vi "BoxExecute.vi"(8 "error in (no error)":errorcluster) -> (0 "error out":errorcluster)   [LabVIEW 2023]
uses:
  <vilib>/Rock Robotics/WPI/ThirdParty/REV Robotics/REVLib/Typedef/Spark MAX Control Type.ctl
  BoxStatesEnum.ctl
  BoxNoteState.ctl
  <vilib>/Rock Robotics/WPI/ThirdParty/JAS_Junk/TrajLib/TypeDef/PID_ERROR_TOLERANCE.ctl
  <vilib>/Rock Robotics/WPI/ThirdParty/JAS_Junk/TrajLib/LinearFilter_LP_BW1_Execute.vi
  <vilib>/Rock Robotics/WPI/ThirdParty/JAS_Junk/TrajLib/VI/BoolCmd_Recv_Internal.vi
  <vilib>/Rock Robotics/WPI/ThirdParty/JAS_Junk/TrajLib/PIDController_AtSetpoint.vi
  <vilib>/Rock Robotics/WPI/ThirdParty/JAS_Junk/TrajLib/PIDController_SetPIDF.vi
  <vilib>/Rock Robotics/WPI/ThirdParty/JAS_Junk/TrajLib/PIDController_SetDerivativeFilter.vi
  <vilib>/Rock Robotics/WPI/ThirdParty/JAS_Junk/TrajLib/PIDController_SetIntegratorRange.vi
  <vilib>/Rock Robotics/WPI/ThirdParty/JAS_Junk/TrajLib/PIDController_SetTolerancePandV.vi
  <vilib>/Rock Robotics/WPI/ThirdParty/JAS_Junk/TrajLib/PIDController_DisableContinousInput.vi
  <vilib>/Rock Robotics/WPI/ThirdParty/JAS_Junk/TrajLib/PIDController_EnableContinousInput.vi
  <vilib>/Rock Robotics/WPI/ThirdParty/JAS_Junk/TrajLib/PIDController_Reset.vi
  <vilib>/Rock Robotics/WPI/ThirdParty/JAS_Junk/TrajLib/PIDController_New.vi
  <vilib>/Rock Robotics/WPI/ThirdParty/JAS_Junk/TrajLib/PIDController_SetOutputLimits.vi
  <vilib>/Rock Robotics/WPI/ThirdParty/JAS_Junk/TrajLib/VI/PIDController_SetIntegratorZone.vi
  <vilib>/Rock Robotics/WPI/ThirdParty/JAS_Junk/TrajLib/SimpleMotorFF_Calculate.vi
  <vilib>/Rock Robotics/WPI/ThirdParty/JAS_Junk/TrajLib/LinearFilter_ResetToValue.vi
  <vilib>/Rock Robotics/WPI/ThirdParty/JAS_Junk/TrajLib/LinearFilter_Calculate.vi
  <vilib>/Rock Robotics/WPI/ThirdParty/JAS_Junk/TrajLib/SlewRateLimiter_New.vi
  <vilib>/Rock Robotics/WPI/ThirdParty/JAS_Junk/TrajLib/SlewRateLimiter_Reset.vi
  <vilib>/Rock Robotics/WPI/ThirdParty/JAS_Junk/TrajLib/SlewRateLimiter_Calculate.vi
  <vilib>/Rock Robotics/WPI/ThirdParty/JAS_Junk/TrajLib/SlewRateLimiter_SetRate.vi
  <vilib>/Rock Robotics/WPI/ThirdParty/JAS_Junk/TrajLib/VI/BoolCmd_ObtainQueue.vi
  <vilib>/Rock Robotics/WPI/ThirdParty/JAS_Junk/TrajLib/PIDController_NewPeriod.vi
  <vilib>/Rock Robotics/WPI/ThirdParty/JAS_Junk/TrajLib/Util_GetTime.vi
  <vilib>/Rock Robotics/SystemInterfaces/NetworkCommunication/NetComm_UsageReport_report.vi
  <vilib>/Rock Robotics/WPI/ThirdParty/JAS_Junk/TrajLib/VI/Util_GetTime_U32.vi
  BoxGlobals.vi
  BoxNetworkingGlobal.vi
  <vilib>/Rock Robotics/WPI/ThirdParty/REV Robotics/REVLib/SubVI/Public/SPARK Get Encoder Status Velocity.vi
  <vilib>/Utility/semaphor.llb/Obtain Semaphore Reference.vi
  <vilib>/Rock Robotics/WPI/ThirdParty/JAS_Junk/TrajLib/Timer_Reset.vi
  <vilib>/Rock Robotics/WPI/ThirdParty/JAS_Junk/TrajLib/Timer_Start.vi
  <vilib>/Rock Robotics/WPI/ThirdParty/JAS_Junk/TrajLib/Timer_Stop.vi
  <vilib>/Rock Robotics/WPI/ThirdParty/JAS_Junk/TrajLib/LinearFilter_LowPassBW1.vi
  <vilib>/Rock Robotics/SystemInterfaces/Utilities/FPGA_UtilitiesRead LocalTime.vi
  <vilib>/Rock Robotics/WPI/ThirdParty/JAS_Junk/TrajLib/VI/Util_GetTime_U64.vi
  <vilib>/Rock Robotics/WPI/ThirdParty/JAS_Junk/TrajLib/Globals/Util_LibraryGlobals.vi
  <vilib>/Rock Robotics/WPI/ThirdParty/JAS_Junk/TrajLib/PIDController_AdvCalculate_FF_Sp_Pv.vi
  <vilib>/Rock Robotics/WPI/ThirdParty/JAS_Junk/TrajLib/Trajectory_Library.lvlib
panel:
  # "Click here to set min"
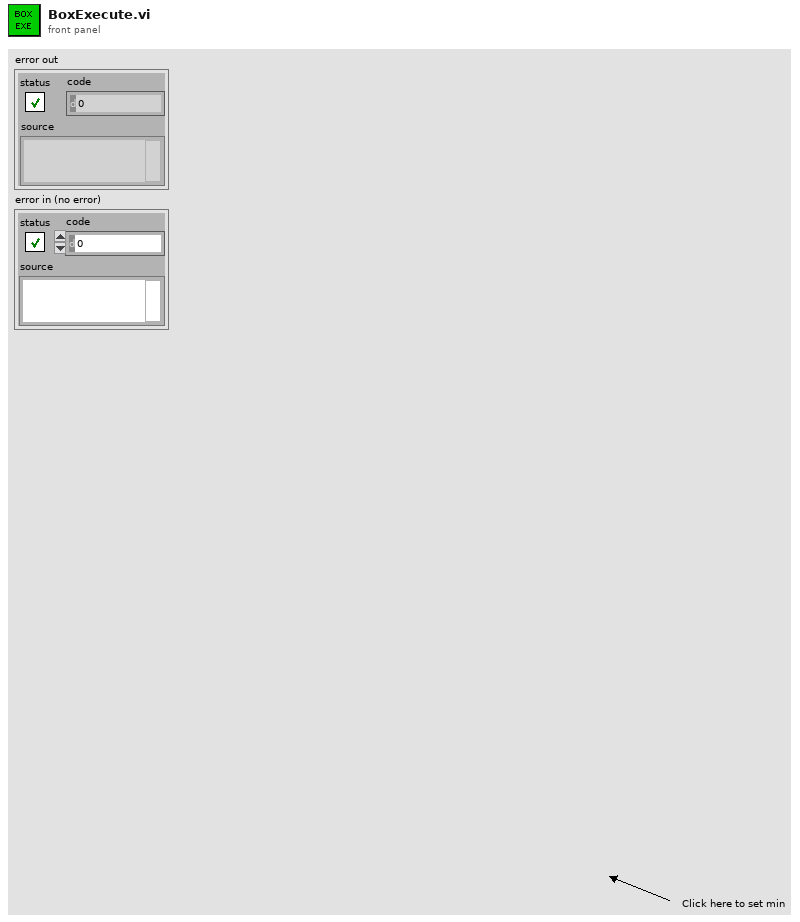
[diagram p1: front panel]
types:
  T1 = typedef "Spark MAX Control Type.ctl" = enum16{"Percent VBus", "Voltage", "Velocity", "Position", "Smart Motion", "Current", "Smart Velocity", "MAXMotion Position", "MAXMotion Velocity"}
  T2 = typedef "BoxStatesEnum.ctl" = enum16{"get input", "start shoot wheels", "up to speed?", "run intake", "have ring?", "stop intake and shooter", "start intake", "pick up ring or  _ sec?", "stop intake", "start source  intake", "pick up note?", "stop intake shooter", "shoot amp", "used note?", "stop amp intake", "initilization", "pre rev"}
  T3 = typedef "BoxNoteState.ctl" = enum16{"note in shooter wheels", "misaligned note", "no note", "have note"}
  T4 = typedef "Trajectory_Library.lvlib/PID_ERROR_TOLERANCE.ctl" = cluster{"PositionTolerance":dbl, "VelocityTolerance":dbl}
  T5 = typedef "WPI_DigitalInputDevRef.ctl" = cluster{"DevStatus":errorcluster, "DIO Channel":T6}
  T6 = typedef "FPGA_DIOChannel.ctl" = enum8{"DIO 0", "DIO 1", "DIO 2", "DIO 3", "DIO 4", "DIO 5", "DIO 6", "DIO 7", "DIO 8", "DIO 9", "DIO MXP 0", "DIO MXP 1", "DIO MXP 2", "DIO MXP 3", "DIO MXP 4", "DIO MXP 5", "DIO MXP 6", "DIO MXP 7", "DIO MXP 8", "DIO MXP 9", "DIO MXP 10", "DIO MXP 11", "DIO MXP 12", "DIO MXP 13", "DIO MXP 14", "DIO MXP 15", "SPI Port CS1", "SPI Port CS2", "SPI Port CS3", "SPI Port MISO", "SPI Port MOSI", "Invalid"}
  T7 = typedef "WPI_MotorControlDeviceRef.ctl" = cluster{"DeviceStatus":errorcluster, "Type":T8, "PWM":cluster{"PWM Channel":T9, "DeadBand":T10}, "CAN":cluster{"Device Number":u8, "SetOutput VI Ref":variant, "GetOutput VI Ref":variant, "Enable VI Ref":variant, "Disable VI Ref":variant, "Data":variant}, "Invert":bool, "DIO PWM":cluster{"PWM \"Enable\" Channel":T9, "DIOChannel":T6, "PWM Rate":dbl}}
  T8 = typedef "WPI_MotorControlType.ctl" = enum16{"PWM", "CAN", "DIO PWM"}
  T9 = typedef "FPGA_DIOPWMChannel.ctl" = enum8{"PWM 0", "PWM 1", "PWM 2", "PWM 3", "PWM 4", "PWM 5", "PWM 6", "PWM 7", "PWM 8", "PWM 9", "PWM MXP 0", "PWM MXP 1", "PWM MXP 2", "PWM MXP 3", "PWM MXP 4", "PWM MXP 5", "PWM MXP 6", "PWM MXP 7", "PWM MXP 8", "PWM MXP 9", "Invalid"}
  T10 = typedef "WPI_PWMDeadband.ctl" = cluster{"Name":string, "maxPositivePwm":i32, "minPositivePwm":i32, "centerPwm":i32, "maxNegativePwm":i32, "minNegativePwm":i32, "angularRange":u16}
  T11 = typedef "Trajectory_Library.lvlib/TIMER.ctl" = cluster{"StartTime":dbl, "Accumulated TIme":dbl, "Running":bool, "semaphore":T12}
  T12 = typedef "Semaphore RefNum" = refnum<k1>
  T13 = typedef "Trajectory_Library.lvlib/SIMPLE_MOTOR_FF.ctl" = cluster{"Ks":dbl, "Kv":dbl, "Ka":dbl, "KnInv":dbl}
  T14 = typedef "Trajectory_Library.lvlib/PID_ADV_LIMITS.ctl" = cluster{"MaxInput":dbl, "MinInput":dbl, "Continuous":bool, "MaxOutput":dbl, "MinOutput":dbl}
  T15 = typedef "Trajectory_Library.lvlib/PID_ADV_TUNING.ctl" = cluster{"Kf":dbl, "Kp":dbl, "Ki":dbl, "Kd":dbl, "MaximumIntegral":dbl, "MinimumIntegral":dbl, "Filter Derivative":bool, "IntegralZone":dbl}
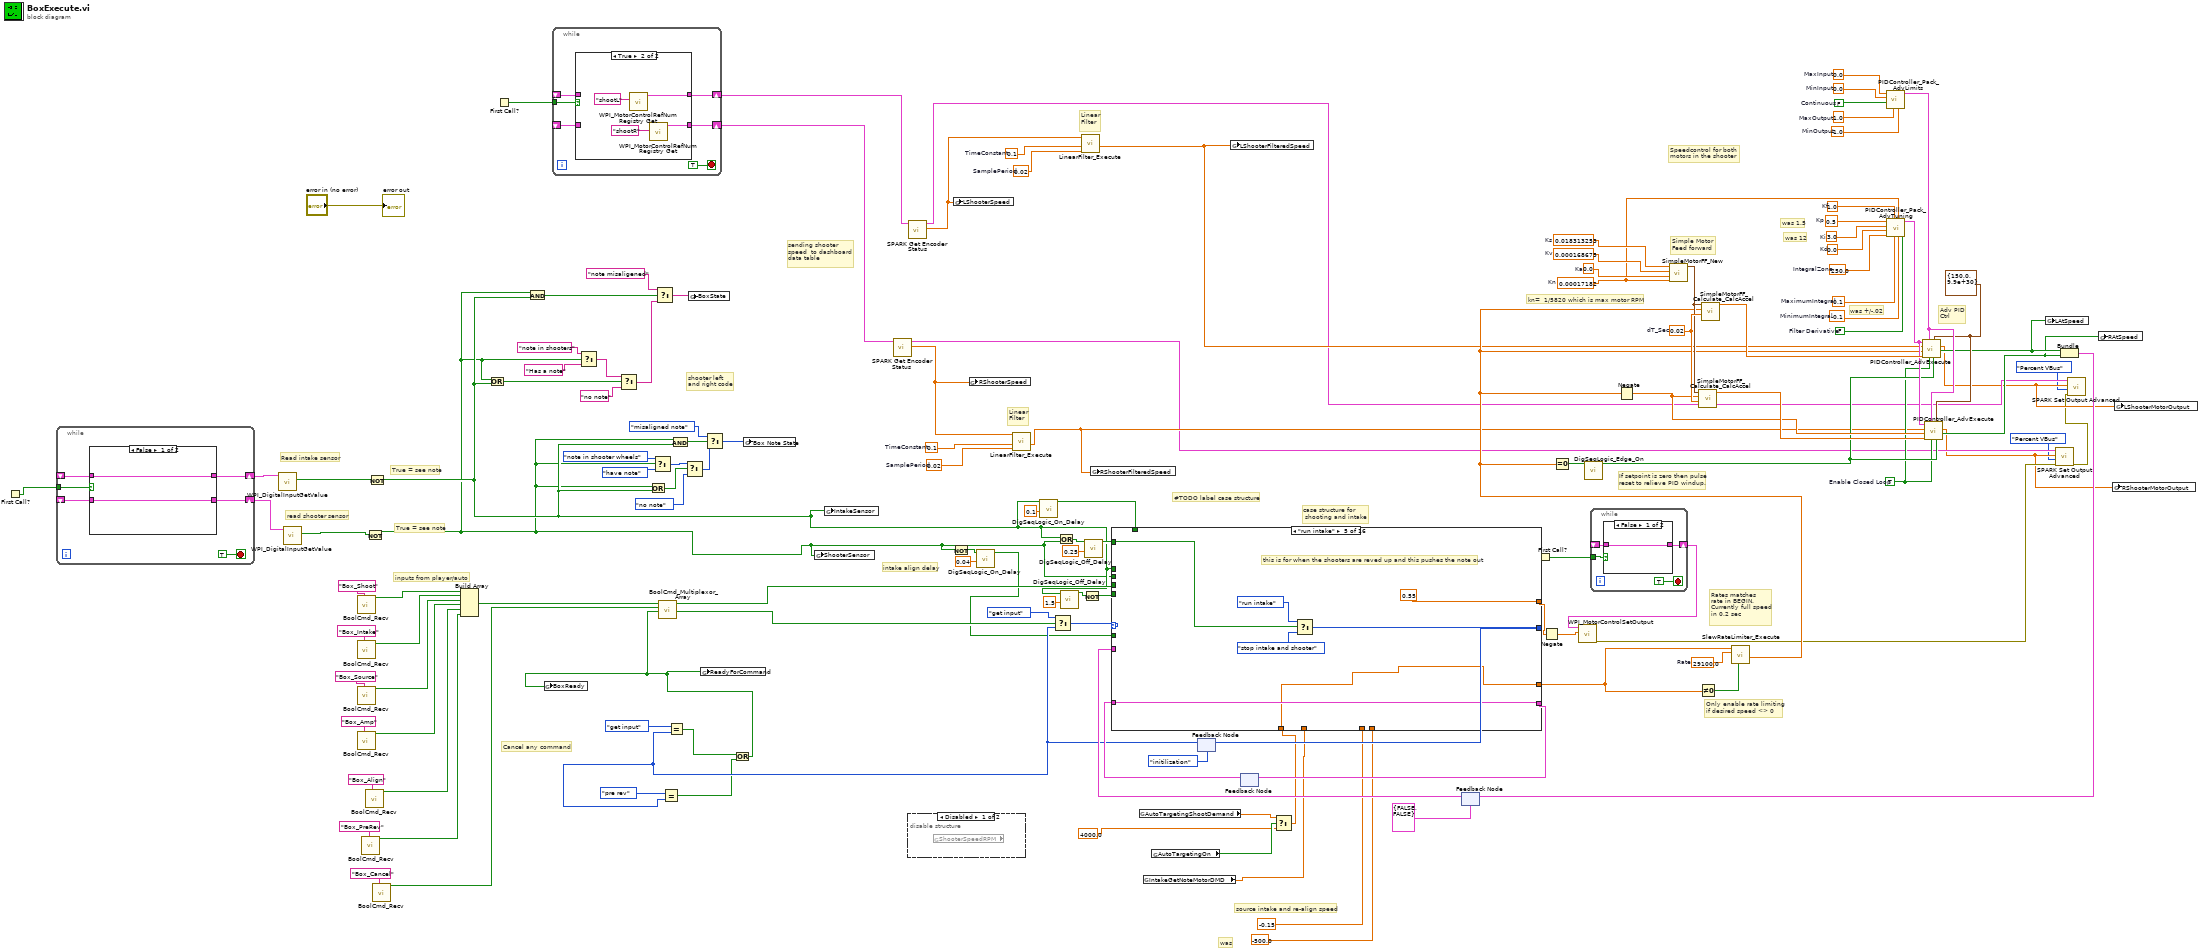
[diagram p0: block diagram]
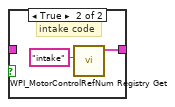
[diagram p3: hidden frame]
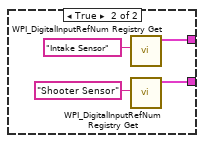
[diagram p4: hidden frame]
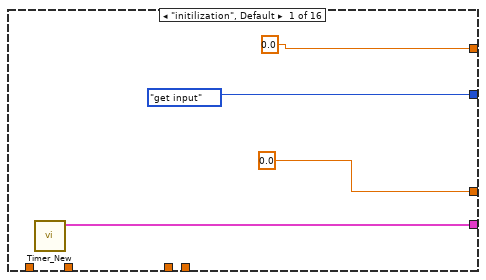
[diagram p6: hidden frame]
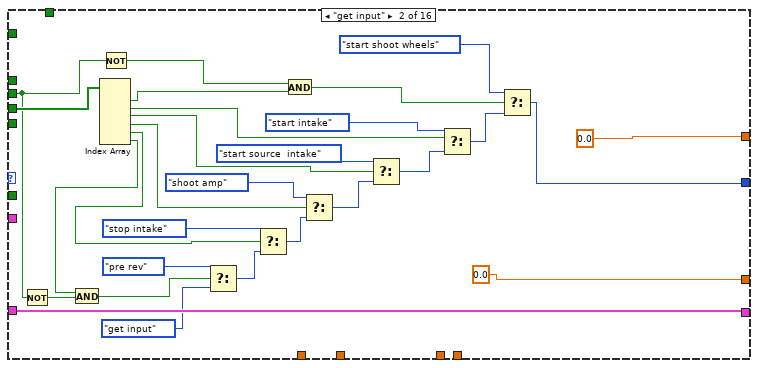
[diagram p7: hidden frame]
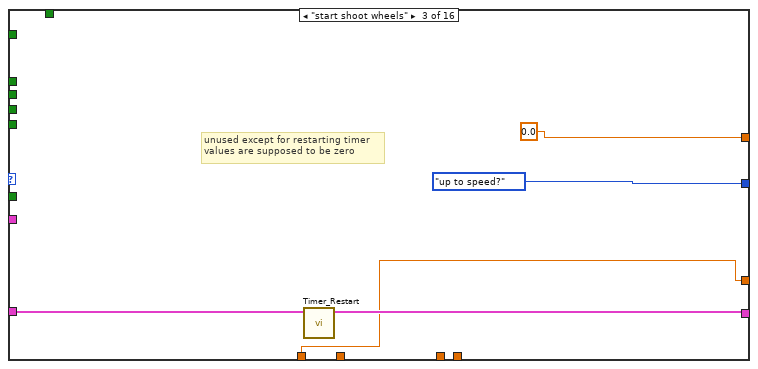
[diagram p8: hidden frame]
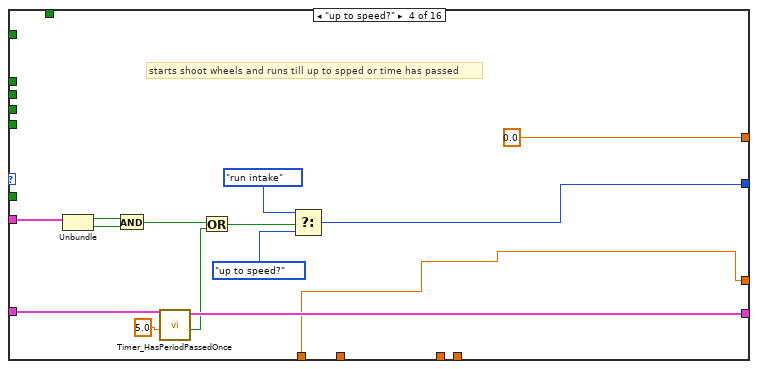
[diagram p9: hidden frame]
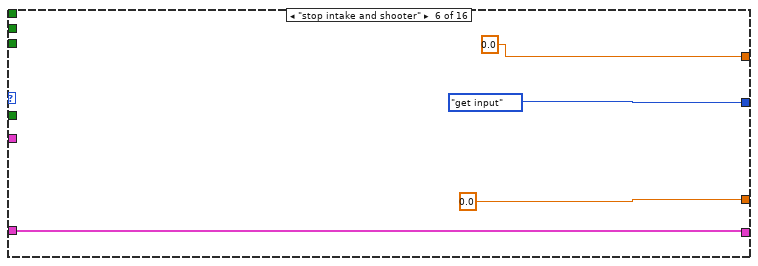
[diagram p10: hidden frame]
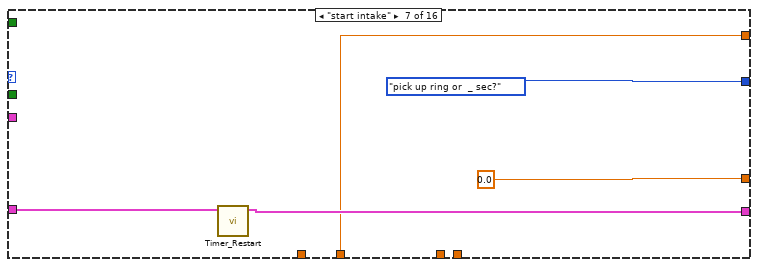
[diagram p11: hidden frame]
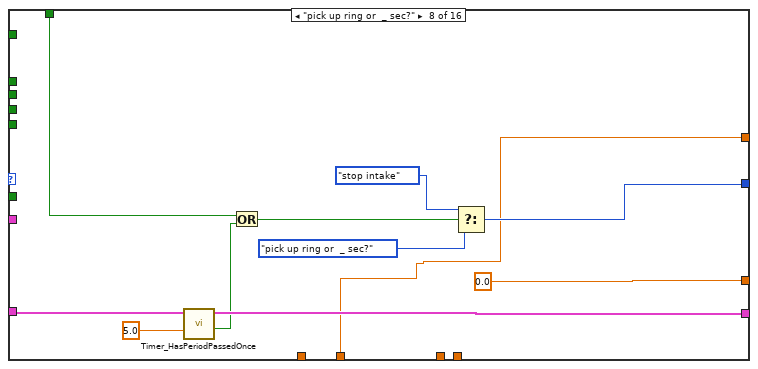
[diagram p12: hidden frame]
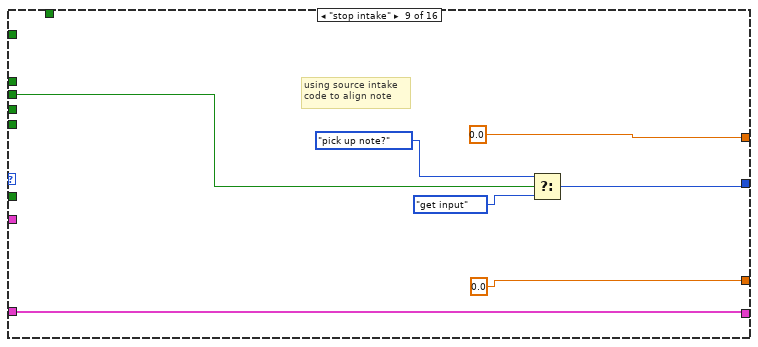
[diagram p13: hidden frame]
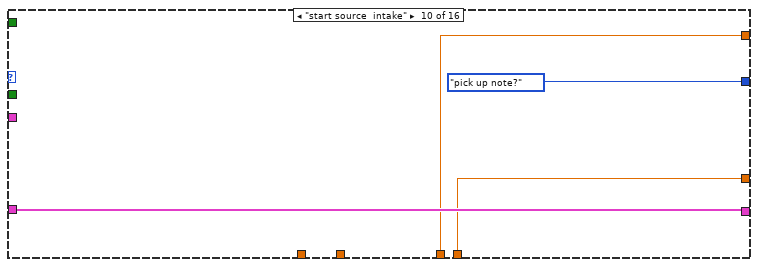
[diagram p14: hidden frame]
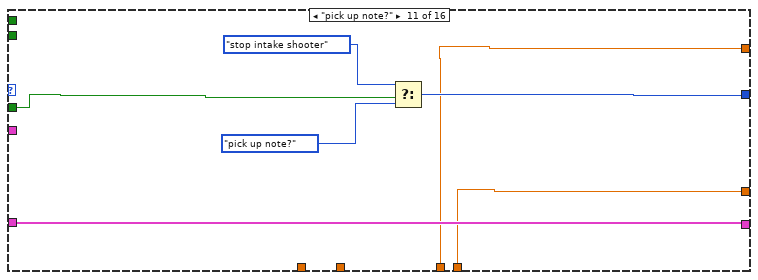
[diagram p15: hidden frame]
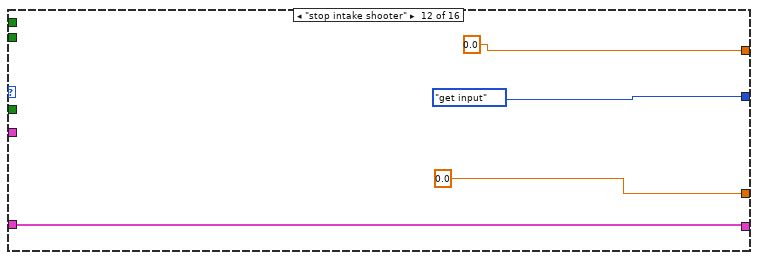
[diagram p16: hidden frame]
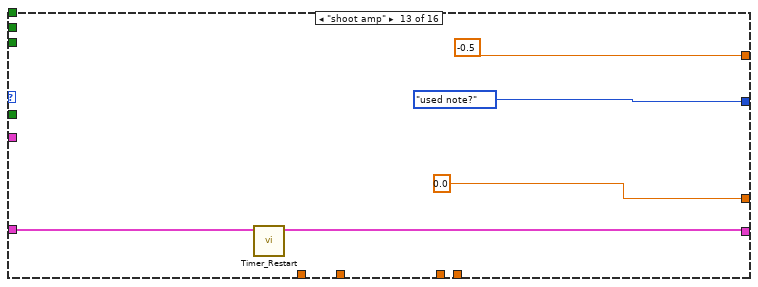
[diagram p17: hidden frame]
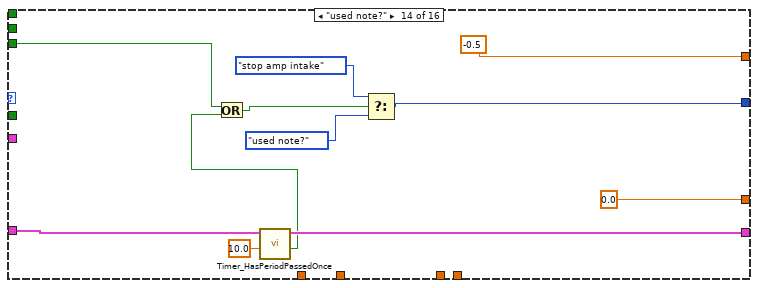
[diagram p18: hidden frame]
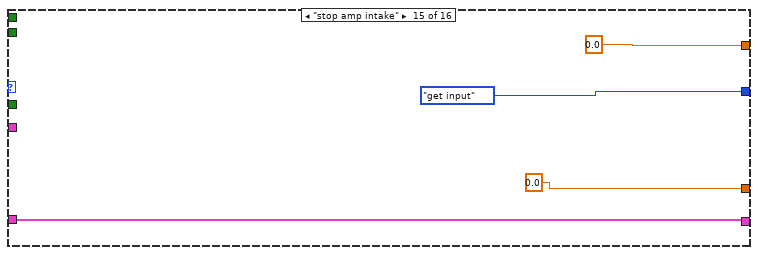
[diagram p19: hidden frame]
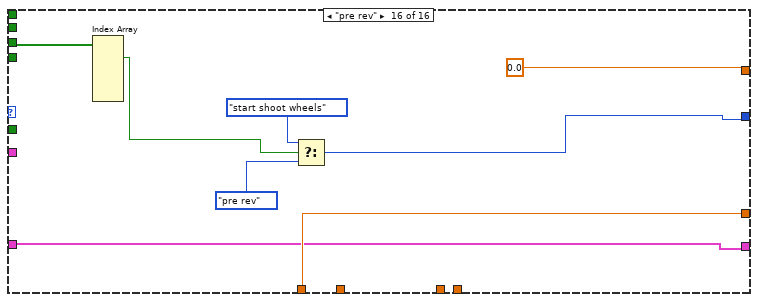
[diagram p20: hidden frame]
diagram:
  w21 = 250.0  # IntegralZone
  w50 = 29100.0  # Rate
  w12 = 0.02  # SamplePeriod
  w13 = 0.1  # TimeConstant
  w85 = 0.02  # SamplePeriod
  w9 = 0.1  # TimeConstant
  w47 = TRUE  # Enable Closed Loop
  w89 = T4 {"PositionTolerance"=150.0, "VelocityTolerance"=9.9e+30} ("PID Error Tolerance")
  w101 = 0.00017182  # Kn
  w104 = 0.018313253  # Ks
  w103 = 0.000168675  # Kv
  w102 = 0.0  # Ka
  w99 = 0.5  # Kp
  w98 = 3.0  # Ki
  w97 = 0.0  # Kd
  w100 = 1.0  # Kf
  w96 = 0.1  # MaximumIntegral
  w95 = -0.1  # MinimumIntegral
  w94 = FALSE  # Filter Derivative
  w108 = 0.0  # MinInput
  w107 = FALSE  # Continuous
  w106 = 1.0  # MaxOutput
  w105 = -1.0  # MinOutput
  w109 = 0.0  # MaxInput
  w93 = 0.02  # dT_Sec
  # "intake align delay"
  # "was"
  # "source intake and re-align speed"
  # "was 12"
  # "was 1.5"
  # "True = see note"
  # "True = see note"
  # "read shooter sensor"
  # "Read intake sensor"
  # "was +/-.02"
  # "If setpoint is zero then pulse\nreset to relieve PID windup."
  # "Rates matches\nrate in BEGIN.  \nCurrently full speed\nin 0.2 sec"
  # "Only enable rate limiting\nif desired speed <> 0"
  # "#TODO label case structure"
  # "inputs from player/auto"
  # "Linear\nFilter"
  # "Linear\nFilter"
  # "Speedcontrol for both \nmotors in the shooter"
  # "Simple Motor\nFeed forward"
  # "Adv PID\nCtrl"
  # "Cancel any command"
  # "kn=  1/5820 which is max motor RPM"
  # "case structure for\n shooting and intake"
  # "sending shooter \nspeed  to dashboard \ndata table"
  # "shooter left \nand right code"
  n1 = First Call?() -> (First Call?: T/F=w45:bool)
  n2 = while {
    tunnel: w45 -> [w137]
    shift-right: [w138] -> w113
    shift-left: _ -> [w136]
    shift-right: [w139] -> w114
    shift-left: _ -> [w135]
    stop <- TRUE stop-if-true
    n3 = case shown="False" w137 {
      tunnel: [w140 w145] -> w139
      tunnel: [w141 w144] -> w138
      tunnel: w136 -> [w141 _]
      tunnel: w135 -> [w140 _]
      frame False {
      }
      frame True {
        n4 = call <vilib>:"WPI_DigitalInputRefNum Registry Get.vi"("refnum name"="Intake Sensor") -> ("DigitalInputDevRef"=w144:T5)  [unwired: 9 in, 1 out]
        n5 = call <vilib>:"WPI_DigitalInputRefNum Registry Get.vi"("refnum name"="Shooter Sensor") -> ("DigitalInputDevRef"=w145:T5)  [unwired: 9 in, 1 out]
      }
    }
  }
  n6 = call <vilib>:"WPI_DigitalInputGetValue.vi"("DigitalInputDevRef"=w113) -> ("Value"=w74:bool)  [unwired: 8 in, 2 out]
  n7 = call <vilib>:"WPI_DigitalInputGetValue.vi"("DigitalInputDevRef"=w114) -> ("Value"=w73:bool)  [unwired: 8 in, 2 out]
  n8 = call <vilib>:"BoolCmd_Recv.vi"("Command Name"="Box_Shoot") -> ("New Request"=w124:bool)  [unwired: 9 in, 1 out]
  n9 = call <vilib>:"BoolCmd_Recv.vi"("Command Name"="Box_Intake") -> ("New Request"=w125:bool)  [unwired: 9 in, 1 out]
  n10 = call <vilib>:"BoolCmd_Recv.vi"("Command Name"="Box_Source") -> ("New Request"=w128:bool)  [unwired: 9 in, 1 out]
  n11 = call <vilib>:"BoolCmd_Recv.vi"("Command Name"="Box_Amp") -> ("New Request"=w129:bool)  [unwired: 9 in, 1 out]
  n12 = call <vilib>:"BoolCmd_Recv.vi"("Command Name"="Box_PreRev") -> ("New Request"=w38:bool)  [unwired: 9 in, 1 out]
  n13 = call <vilib>:"BoolCmd_Recv.vi"("Command Name"="Box_Align") -> ("New Request"=w53:bool)  [unwired: 9 in, 1 out]
  n14 = Not(x=w73) -> (.not. x?=w18:bool)
  n15 = Not(x=w74) -> (.not. x?=w30:bool)
  n16 = call <vilib>:"BoolCmd_Recv.vi"("Command Name"="Box_Cancel") -> ("New Request"=w122:bool)  [unwired: 9 in, 1 out]
  n17 = Build Array(w124, w125, w128, w129, w53, w38) -> (w123:bool[])
  n18 = Or(x=w18, y=w30) -> (x .or. y?=w81:bool)
  n19 = First Call?() -> (First Call?: T/F=w46:bool)
  n20 = And(x=w18, y=w30) -> (x .and. y?=w82:bool)
  n21 = while {
    tunnel: w46 -> [w149]
    shift-right: [w151] -> w15
    shift-left: _ -> [w147]
    shift-right: [w150] -> w11
    shift-left: _ -> [w146]
    stop <- TRUE stop-if-true
    n22 = case shown="True" w149 {
      tunnel: [w153 w155] -> w151
      tunnel: [w152 w154] -> w150
      tunnel: w147 -> [w153 _]
      tunnel: w146 -> [w152 _]
      frame False {
      }
      frame True {
        n23 = call <vilib>:"WPI_MotorControlRefNum Registry Get.vi"("refnum name"="shootL") -> ("MotorControlDevRef"=w155:T7)  [unwired: 9 in, 1 out]
        n24 = call <vilib>:"WPI_MotorControlRefNum Registry Get.vi"("refnum name"="shootR") -> ("MotorControlDevRef"=w154:T7)  [unwired: 9 in, 1 out]
      }
    }
  }
  n25 = Select(t="note in shooters", s=w18, f="Has a note") -> (s? t:f=w80:string)
  n26 = Select(t=w80, s=w81, f="no note") -> (s? t:f=w78:string)
  n27 = Or(x=w18, y=w30) -> (x .or. y?=w71:bool)
  n28 = Select(t=BoxNoteState."note in shooter wheels" ("Box Note State"), s=w18, f=BoxNoteState."have note" ("Box Note State")) -> (s? t:f=w70:T3)
  n29 = Select(t="note misaligened", s=w82, f=w78) -> (s? t:f=w29:string)
  n30 = And(x=w18, y=w30) -> (x .and. y?=w72:bool)
  n31 = Select(t=w70, s=w71, f=BoxNoteState."no note" ("Box Note State")) -> (s? t:f=w69:T3)
  n32 = global write "BoxNetworkingGlobal.vi" "BoxState"(w29) -> ()
  n33 = Select(t=BoxNoteState."misaligned note" ("Box Note State"), s=w72, f=w69) -> (s? t:f=w64:T3)
  n34 = global write "BoxGlobals.vi" "Box Note State"(w64) -> ()
  n35 = global write "BoxNetworkingGlobal.vi" "ShooterSensor"(w18) -> ()
  n36 = global write "BoxNetworkingGlobal.vi" "IntakeSensor"(w30) -> ()
  n37 = call-poly <vilib>:"SPARK Get Encoder Status.vi"("MotorControlDevRef in"=w11) -> ("Sensor Velocity"=w10:dbl, "MotorControlDevRef out"=w5:T7)  [unwired: 7 in, 2 out]
  n38 = disable-structure shown="Disabled" {
    frame Disabled {
      n39 = global read "BoxGlobals.vi" "ShooterSpeedRPM"() -> ()  [unwired: 1 out]
    }
    frame Enabled {
    }
  }
  n40 = call-poly <vilib>:"SPARK Get Encoder Status.vi"("MotorControlDevRef in"=w15) -> ("Sensor Velocity"=w14:dbl, "MotorControlDevRef out"=w8:T7)  [unwired: 7 in, 2 out]
  n41 = Not(x=w18) -> (.not. x?=w20:bool)
  n42 = global write "BoxNetworkingGlobal.vi" "LShooterSpeed"(w14) -> ()
  n43 = global write "BoxNetworkingGlobal.vi" "RShooterSpeed"(w10) -> ()
  n44 = call <vilib>:"DigSeqLogic_On_Delay.vi"("Delay"=0.04, "Input"=w20) -> ("Output"=w17:bool)  [unwired: 8 in, 1 out]
  n45 = call-poly <vilib>:"LinearFilter_Execute.vi"("SamplePeriod"=w85, "TimeConstant"=w9, "Input"=w10) -> ("Output"=w33:dbl)  [unwired: 8 in]
  n46 = call <vilib>:"DigSeqLogic_On_Delay.vi"("Delay"=0.1 ("On Delay Time\nSeconds"), "Input"=w30) -> ("Output"=w40:bool)  [unwired: 8 in, 1 out]
  n47 = Or(x=w30, y=w18) -> (x .or. y?=w59:bool)
  n48 = call <vilib>:"DigSeqLogic_Off_Delay.vi"("Delay"=1.5 ("Off Delay Tme\nSeconds"), "Input"=w30) -> ("Output"=w56:bool)  [unwired: 8 in, 1 out]
  n49 = call-poly <vilib>:"LinearFilter_Execute.vi"("SamplePeriod"=w12, "TimeConstant"=w13, "Input"=w14) -> ("Output"=w34:dbl)  [unwired: 8 in]
  n50 = Not(x=w56) -> (.not. x?=w55:bool)
  n51 = call <vilib>:"DigSeqLogic_Off_Delay.vi"("Delay"=0.25 ("Off Delay Tme\nSeconds"), "Input"=w59) -> ("Output"=w58:bool)  [unwired: 8 in, 1 out]
  n52 = global write "BoxNetworkingGlobal.vi" "RShooterFilteredSpeed"(w33) -> ()
  n53 = global read "BoxGlobals.vi" "AutoTargetingShootDemand"() -> (w37:dbl)
  n54 = global read "BoxGlobals.vi" "IntakeGetNoteMotorDMD"() -> (w43:dbl)
  n55 = global read "BoxGlobals.vi" "AutoTargetingOn"() -> (w36:bool)
  n56 = feedback #1(BoxStatesEnum."initilization") -> (w25:T2)
  n57 = Equal?(x=BoxStatesEnum."pre rev" ("Box states"), y=w25) -> (x = y?=w24:bool)
  n58 = Equal?(x=BoxStatesEnum."get input" ("Box states"), y=w25) -> (x = y?=w23:bool)
  n59 = Or(x=w23, y=w24) -> (x .or. y?=w22:bool)
  n60 = global write "BoxNetworkingGlobal.vi" "BoxReady"(w22) -> ()
  n61 = call <vilib>:"BoolCmd_Multiplexor_Array.vi"("Ready"=w22, "Command Cancel"=w122, "Commands"=w123) -> ("Do Cancel"=w116:bool, "Do Command"=w118:bool[])  [unwired: 7 in]
  n62 = global write "BoxGlobals.vi" "ReadyForCommand"(w22) -> ()
  n63 = Select(t=BoxStatesEnum."get input" ("Box states"), s=w116, f=w25) -> (s? t:f=w117:T2)
  n64 = global write "BoxNetworkingGlobal.vi" "LShooterFilteredSpeed"(w34) -> ()
  n65 = feedback #2() -> (w83:T11)  [unwired: 1 in]
  n66 = Select(t=w37, s=w36, f=4000.0) -> (s? t:f=w35:dbl)
  n67 = feedback #3(cluster{bool, bool} {FALSE, FALSE}) -> (w131:cluster{bool, bool})
  n68 = case shown="\"run intake\"" w117 {
    tunnel: [BoxStatesEnum."get input" ("Box states") w183 BoxStatesEnum."up to speed?" ("Box states") w203 w212 BoxStatesEnum."get input" ("Box states") BoxStatesEnum."pick up ring or  _ sec?" ("Box states") w232 w239 BoxStatesEnum."pick up note?" ("Box states") w250 BoxStatesEnum."get input" ("Box states") BoxStatesEnum."used note?" ("Box states") w269 BoxStatesEnum."get input" ("Box states") w282] -> w132
    tunnel: w131 -> [_ _ _ w206 _ _ _ _ _ _ _ _ _ _ _ _]
    tunnel: [0.0 0.0 w190 w195 w209 0.0 0.0 0.0 0.0 w243 w248 0.0 0.0 0.0 0.0 w283] -> w48
    tunnel: [0.0 0.0 0.0 0.0 0.55 0.0 w220 w226 0.0 w244 w249 0.0 -0.5 -0.5 0.0 0.0] -> w61
    tunnel: w118 -> [_ w188 _ _ _ _ _ _ _ _ _ _ _ _ _ w280]
    tunnel: w30 -> [_ _ _ _ _ _ _ _ _ _ _ _ _ _ _ _]
    tunnel: w18 -> [_ w165 _ _ _ _ _ _ w236 _ _ _ _ _ _ _]
    tunnel: [w158 w175 w191 w200 w211 w216 w222 w228 w240 w245 w253 w254 w258 w267 w274 w281] -> w84
    tunnel: w83 -> [_ w175 w192 w201 w211 w216 w221 w230 w240 w245 w253 w254 w259 w268 w274 w281]
    tunnel: w58 -> [_ _ _ _ w210 _ _ _ _ _ _ _ _ _ _ _]
    tunnel: w55 -> [_ _ _ _ _ _ _ _ _ _ _ _ _ w263 _ _]
    tunnel: w35 -> [_ _ w190 w195 w209 _ _ _ _ _ _ _ _ _ _ w283]
    tunnel: w43 -> [_ _ _ _ _ _ w220 w226 _ _ _ _ _ _ _ _]
    tunnel: w40 -> [_ _ _ _ _ _ _ w225 _ _ _ _ _ _ _ _]
    tunnel: -0.15 -> [_ _ _ _ _ _ _ _ _ w244 w249 _ _ _ _ _]
    tunnel: -500.0 -> [_ _ _ _ _ _ _ _ _ w243 w248 _ _ _ _ _]
    tunnel: w17 -> [_ _ _ _ _ _ _ _ _ _ w247 _ _ _ _ _]
    frame "initilization", Default {
      n69 = call <vilib>:"Timer_New.vi"() -> ("TIMER"=w158:T11)  [unwired: 11 in]
    }
    frame "get input" {
      n70 = Not(x=w165) -> (.not. x?=w163:bool)
      n71 = Index Array(array=w188) -> (element #1=w173:bool, element #2=w180:bool, element #3=w179:bool, element #4=w178:bool, element #5=w169:bool, element #6=w164:bool)  [unwired: 6 in]
      n72 = And(x=w164, y=w163) -> (x .and. y?=w162:bool)
      n73 = Not(x=w165) -> (.not. x?=w172:bool)
      n74 = Select(t=BoxStatesEnum."pre rev" ("Box states"), s=w162, f=BoxStatesEnum."get input" ("Box states")) -> (s? t:f=w168:T2)
      n75 = Select(t=BoxStatesEnum."stop intake" ("Box states"), s=w169, f=w168) -> (s? t:f=w171:T2)
      n76 = And(x=w172, y=w173) -> (x .and. y?=w174:bool)
      n77 = Select(t=BoxStatesEnum."shoot amp" ("Box states"), s=w178, f=w171) -> (s? t:f=w184:T2)
      n78 = Select(t=BoxStatesEnum."start source  intake", s=w179, f=w184) -> (s? t:f=w185:T2)
      n79 = Select(t=BoxStatesEnum."start intake" ("Box states"), s=w180, f=w185) -> (s? t:f=w186:T2)
      n80 = Select(t=BoxStatesEnum."start shoot wheels" ("Box states"), s=w174, f=w186) -> (s? t:f=w183:T2)
    }
    frame "start shoot wheels" {
      # "unused except for restarting timer\nvalues are supposed to be zero"
      n81 = call <vilib>:"Timer_Restart.vi"("in Timer"=w192) -> ("out Timer"=w191:T11)  [unwired: 10 in]
    }
    frame "up to speed?" {
      # "starts shoot wheels and runs till up to spped or time has passed"
      n82 = Unbundle(w206) -> (w205:bool, w204:bool)
      n83 = And(x=w205, y=w204) -> (x .and. y?=w198:bool)
      n84 = call <vilib>:"Timer_HasPeriodPassedOnce.vi"("Period"=5.0, "in Timer"=w201) -> ("Expired"=w196:bool, "out Timer"=w200:T11)  [unwired: 7 in, 1 out]
      n85 = Or(x=w198, y=w196) -> (x .or. y?=w197:bool)
      n86 = Select(t=BoxStatesEnum."run intake" ("Box states"), s=w197, f=BoxStatesEnum."up to speed?" ("Box states")) -> (s? t:f=w203:T2)
    }
    frame "run intake" {
      # "this is for when the shooters are reved up and this pushes the note out"
      n87 = Select(t=BoxStatesEnum."run intake" ("Box states"), s=w210, f=BoxStatesEnum."stop intake and shooter" ("Box states")) -> (s? t:f=w212:T2)
    }
    frame "stop intake and shooter" {
    }
    frame "start intake" {
      n88 = call <vilib>:"Timer_Restart.vi"("in Timer"=w221) -> ("out Timer"=w222:T11)  [unwired: 10 in]
    }
    frame "pick up ring or  _ sec?" {
      n89 = call <vilib>:"Timer_HasPeriodPassedOnce.vi"("Period"=5.0, "in Timer"=w230) -> ("Expired"=w227:bool, "out Timer"=w228:T11)  [unwired: 7 in, 1 out]
      n90 = Or(x=w225, y=w227) -> (x .or. y?=w231:bool)
      n91 = Select(t=BoxStatesEnum."stop intake" ("Box states"), s=w231, f=BoxStatesEnum."pick up ring or  _ sec?" ("Box states")) -> (s? t:f=w232:T2)
    }
    frame "stop intake" {
      # "using source intake \ncode to align note"
      n92 = Select(t=BoxStatesEnum."pick up note?" ("Box states"), s=w236, f=BoxStatesEnum."get input" ("Box states")) -> (s? t:f=w239:T2)
    }
    frame "start source  intake" {
    }
    frame "pick up note?" {
      n93 = Select(t=BoxStatesEnum."stop intake shooter" ("Box states"), s=w247, f=BoxStatesEnum."pick up note?" ("Box states")) -> (s? t:f=w250:T2)
    }
    frame "stop intake shooter" {
    }
    frame "shoot amp" {
      n94 = call <vilib>:"Timer_Restart.vi"("in Timer"=w259) -> ("out Timer"=w258:T11)  [unwired: 10 in]
    }
    frame "used note?" {
      n95 = call <vilib>:"Timer_HasPeriodPassedOnce.vi"("Period"=10.0, "in Timer"=w268) -> ("Expired"=w265:bool, "out Timer"=w267:T11)  [unwired: 7 in, 1 out]
      n96 = Or(x=w263, y=w265) -> (x .or. y?=w264:bool)
      n97 = Select(t=BoxStatesEnum."stop amp intake" ("Box states"), s=w264, f=BoxStatesEnum."used note?" ("Box states")) -> (s? t:f=w269:T2)
    }
    frame "stop amp intake" {
    }
    frame "pre rev" {
      n98 = Index Array(array=w280) -> (element #1=w278:bool)  [unwired: 6 in, 5 out]
      n99 = Select(t=BoxStatesEnum."start shoot wheels" ("Box states"), s=w278, f=BoxStatesEnum."pre rev" ("Box states")) -> (s? t:f=w282:T2)
    }
  }
  n100 = feedback-in #1(w132) -> ()
  n101 = feedback-in #2(w84) -> ()
  n102 = First Call?() -> (First Call?: T/F=w44:bool)
  n103 = Negate(x=w61) -> (-x=w62:dbl)
  n104 = while {
    tunnel: w44 -> [w288]
    shift-right: [w289] -> w130
    shift-left: _ -> [w286]
    stop <- TRUE stop-if-true
    n105 = case shown="False" w288 {
      tunnel: [w290 w291] -> w289
      tunnel: w286 -> [w290 _]
      frame False {
      }
      frame True {
        # "intake code"
        n106 = call <vilib>:"WPI_MotorControlRefNum Registry Get.vi"("refnum name"="intake") -> ("MotorControlDevRef"=w291:T7)  [unwired: 9 in, 1 out]
      }
    }
  }
  n107 = call <vilib>:"WPI_MotorControlSetOutput.vi"("Output"=w62, "MotorControlDevRef"=w130) -> ("error out"=w4:errorcluster)  [unwired: 7 in, 2 out]
  n108 = call <vilib>:"SimpleMotorFF_New.vi"("Kn"=w101, "Ka"=w102, "Kv"=w103, "Ks"=w104) -> ("SIMPLE_MOTOR_FF"=w92:T13)  [unwired: 7 in]
  n109 = Not Equal To 0?(x=w48) -> (x != 0?=w49:bool)
  n110 = call <vilib>:"SlewRateLimiter_Execute.vi"("Enable"=w49, "PositiveRate"=w50, "Input"=w48) -> ("Output"=w42:dbl)  [unwired: 7 in, 1 out]
  n111 = Equal To 0?(x=w42) -> (x = 0?=w52:bool)
  n112 = call <vilib>:"DigSeqLogic_Edge_On.vi"("Input"=w52) -> ("On Edge"=w51:bool)  [unwired: 10 in]
  n113 = Negate(x=w42) -> (-x=w86:dbl)
  n114 = call <vilib>:"SimpleMotorFF_Calculate_CalcAccel.vi"("dT_Sec"=w93, "VelSp"=w86, "SIMPLE_MOTOR_FF"=w92) -> ("FeedForward"=w88:dbl)  [unwired: 8 in]
  n115 = call <vilib>:"SimpleMotorFF_Calculate_CalcAccel.vi"("dT_Sec"=w93, "VelSp"=w42, "SIMPLE_MOTOR_FF"=w92) -> ("FeedForward"=w110:dbl)  [unwired: 8 in]
  n116 = call <vilib>:"PIDController_Pack_AdvLimits.vi"("MinOutput"=w105, "MaxOutput"=w106, "Continuous"=w107, "MinInput"=w108, "MaxInput"=w109) -> ("Adv PID Limits"=w90:T14)  [unwired: 6 in]
  n117 = call <vilib>:"PIDController_Pack_AdvTuning.vi"("Filter Derivative"=w94, "MinimumIntegral"=w95, "Kn"=w101, "MaximumIntegral"=w96, "Kf"=w100, "IntegralZone"=w21, "Kd"=w97, "Ki"=w98, "Kp"=w99) -> ("Adv PID Tuning"=w91:T15)  [unwired: 2 in]
  n118 = call <vilib>:"PIDController_AdvExecute.vi"("Reset"=w51, "PID Error Tolerance"=w89, "Auto"=w47, "Adv PID Limits"=w90, "FF-FeedForward"=w110, "SP-SetPoint"=w42, "PV-Measurement"=w34, "Adv PID Tuning"=w91) -> ("AtSetpoint"=w32:bool, "CO-ControlOutput"=w7:dbl)  [unwired: 1 in, 1 out]
  n119 = call <vilib>:"PIDController_AdvExecute.vi"("Reset"=w51, "PID Error Tolerance"=w89, "Auto"=w47, "Adv PID Limits"=w90, "FF-FeedForward"=w88, "SP-SetPoint"=w86, "PV-Measurement"=w33, "Adv PID Tuning"=w91) -> ("AtSetpoint"=w31:bool, "CO-ControlOutput"=w2:dbl)  [unwired: 1 in, 1 out]
  n120 = global write "BoxNetworkingGlobal.vi" "LAtSpeed"(w32) -> ()
  n121 = call <vilib>:"SPARK Set Output Advanced.vi"("error in (no error)"=w4, "Control Mode"=Spark_MAX_Control_Type."Percent VBus", "Setpoint"=w2, "MotorControlDevRef"=w5) -> ("error out"=w3:errorcluster)  [unwired: 6 in, 1 out]
  n122 = Bundle("AtSetpoint"=w32, "AtSetpoint"=w31) -> (w87:cluster{"AtSetpoint":bool, "AtSetpoint":bool})  [unwired: 1 in]
  n123 = feedback-in #3(w87) -> ()
  n124 = call <vilib>:"SPARK Set Output Advanced.vi"("error in (no error)"=w3, "Control Mode"=Spark_MAX_Control_Type."Percent VBus", "Setpoint"=w7, "MotorControlDevRef"=w8) -> ()  [unwired: 6 in, 2 out]
  n125 = global write "BoxNetworkingGlobal.vi" "RAtSpeed"(w31) -> ()
  n126 = global write "BoxNetworkingGlobal.vi" "RShooterMotorOutput"(w2) -> ()
  n127 = global write "BoxNetworkingGlobal.vi" "LShooterMotorOutput"(w7) -> ()
  "error out" <- "error in (no error)"
